vi "Ramp Vector Double, New.vi"(1 "step (1.0)":dbl=1.0, 2 "nelem":i32=5, 3 "start (0.0)":dbl format="%#.6g") -> (0 "ramp":dbl[](array[numeric]))   [LabVIEW 2010]
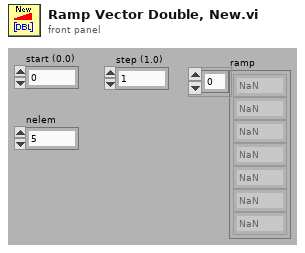
[diagram p1: front panel]
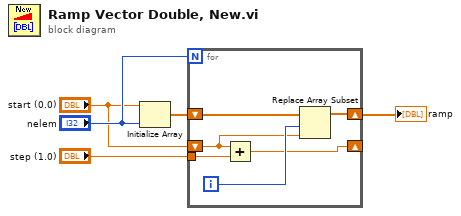
[diagram p0: block diagram]
diagram:
  n1 = Initialize Array("start (0.0)", "nelem") -> (w5:dbl[])
  n2 = for {
    N: "nelem" -> [_]
    shift-right: [w11] -> w4
    shift-left: w5 -> [w10]
    shift-right: [w7] -> _
    shift-left: "start (0.0)" -> [w6]
    tunnel: "step (1.0)" -> [w8]
    i -> [w9]
    n3 = Add(x=w6, y=w8) -> (x+y=w7:dbl)
    n4 = Replace Array Subset(array=w10, new element=w6, index=w9) -> (w11:dbl[])
  }
  "ramp" <- w4
